vi "WPI_CANJaguar_GetVersion.vi"(8 "error in (no error)":errorcluster, 11 "CAN Jaguar Ref":T1={"DeviceStatus"={"status"=FALSE, "code"=0, "source"=""}, "Type"=enum."PWM", "PWM"={"PWM Channel"=enum."PWM 1", "DeadBand"={"Name"="", "maxPositivePwm"=0, "minPositivePwm"=0, "centerPwm"=0, "maxNegativePwm"=0, "minNegativePwm"=0, "angularRange"=0}}, "CAN"={"Device Number"=0, "SetOutput VI Ref"=variant(enum8{"Percent VBus", "Current", "Speed", "Position", "Voltage"} enum."Percent VBus"), "GetOutput VI Ref"=variant(refnum<k1> refnum), "Enable VI Ref"=variant(dbl 12.0), "Disable VI Ref"=variant(enum8{"Percent VBus", "Speed", "Position", "Slave", "Unchanged / Invalid", "Voltage Compensation", "Current", "Motion Profile"} enum."Percent VBus"), "Data"=variant}, "Invert"=FALSE}) -> (0 "error out":errorcluster, 1 "Hardware Version":u8, 2 "Firmware Version":u32, 3 "CAN Jaguar Ref Out":T1={"DeviceStatus"={"status"=FALSE, "code"=0, "source"=""}, "Type"=enum."PWM", "PWM"={"PWM Channel"=enum."PWM 1", "DeadBand"={"Name"="", "maxPositivePwm"=0, "minPositivePwm"=0, "centerPwm"=0, "maxNegativePwm"=0, "minNegativePwm"=0, "angularRange"=0}}, "CAN"={"Device Number"=0, "SetOutput VI Ref"=variant(enum8{"Percent VBus", "Current", "Speed", "Position", "Voltage"} enum."Percent VBus"), "GetOutput VI Ref"=variant(refnum<k1> refnum), "Enable VI Ref"=variant(dbl 12.0), "Disable VI Ref"=variant(enum8{"Percent VBus", "Speed", "Position", "Slave", "Unchanged / Invalid", "Voltage Compensation", "Current", "Motion Profile"} enum."Percent VBus"), "Data"=variant}, "Invert"=FALSE})   [LabVIEW 2016]
uses:
  <vilib>/Rock Robotics/WPI/MotorControl/WPI_MotorControlDeviceRef.ctl
  <vilib>/Rock Robotics/WPI/MotorControl/WPI_MotorControlType.ctl
  <vilib>/Rock Robotics/SystemInterfaces/DIO/FPGA_DIOPWMChannel.ctl
  <vilib>/Rock Robotics/WPI/PWM/WPI_PWMDeadband.ctl
  <vilib>/Rock Robotics/WPI/ThirdParty/CanMotor/CAN Jaguar/SubVIs/WPI_CAN_SystemMessageIDs.ctl
  <vilib>/Rock Robotics/WPI/ThirdParty/CanMotor/CAN Jaguar/SubVIs/WPI_CAN_UpdateMessageIDs.ctl
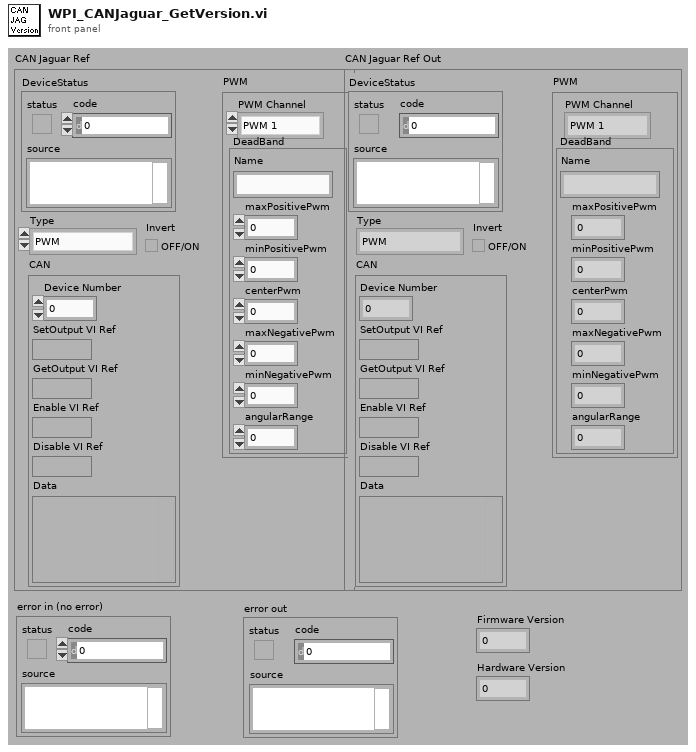
[diagram p1: front panel]
types:
  T1 = typedef "WPI_MotorControlDeviceRef.ctl" = cluster{"DeviceStatus":errorcluster, "Type":T2, "PWM":cluster{"PWM Channel":T3, "DeadBand":T4}, "CAN":cluster{"Device Number":u8, "SetOutput VI Ref":variant, "GetOutput VI Ref":variant, "Enable VI Ref":variant, "Disable VI Ref":variant, "Data":variant}, "Invert":bool}
  T2 = typedef "WPI_MotorControlType.ctl" = enum16{"PWM", "CAN"}
  T3 = typedef "FPGA_DIOPWMChannel.ctl" = enum8{"PWM 0", "PWM 1", "PWM 2", "PWM 3", "PWM 4", "PWM 5", "PWM 6", "PWM 7", "PWM 8", "PWM 9", "PWM MXP 0", "PWM MXP 1", "PWM MXP 2", "PWM MXP 3", "PWM MXP 4", "PWM MXP 5", "PWM MXP 6", "PWM MXP 7", "PWM MXP 8", "PWM MXP 9", "Invalid"}
  T4 = typedef "WPI_PWMDeadband.ctl" = cluster{"Name":string, "maxPositivePwm":i32, "minPositivePwm":i32, "centerPwm":i32, "maxNegativePwm":i32, "minNegativePwm":i32, "angularRange":u16}
  T5 = enum16{"big-endian, network order", "native, host order", "little-endian"}
  T6 = typedef "WPI_CAN_SystemMessageIDs.ctl" = u32
  T7 = typedef "WPI_CAN_UpdateMessageIDs.ctl" = u32
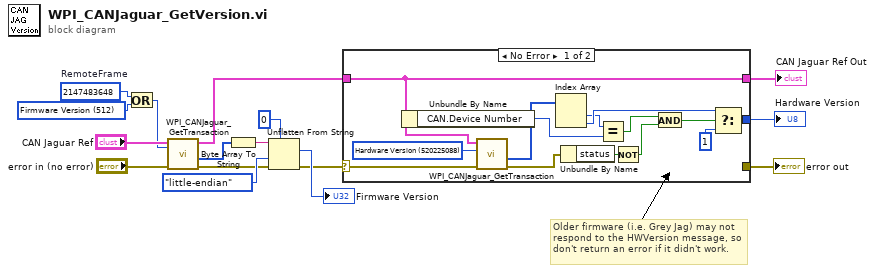
[diagram p0: block diagram]
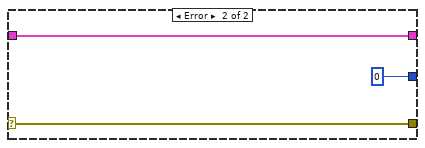
[diagram p2: hidden frame]
diagram:
  w1 = u32 2147483648  # RemoteFrame
  w8 = T6 512 items=["Device Assignment"=128, "Device Query"=192, "Sync Update"=384, "Firmware Update"=448, "Firmware Version"=512, "Enumerate"=576] ("CAN System Message IDs")
  # "Older firmware (i.e. Grey Jag) may not respond to the HWVersion message, so don't return an error if it didn't work."
  n1 = Or(x=w1, y=w8) -> (x .or. y?=w2:T6)
  n2 = call <vilib>:"WPI_CANJaguar_GetTransaction.vi"("error in"="error in (no error)", "Message ID"=w2, "CAN Jaguar Ref"="CAN Jaguar Ref") -> ("error out"=w6:errorcluster, "Data Out"=w3:u8[], "CAN Jaguar Ref Out"=w5:T1)  [unwired: 6 out]
  n3 = Byte Array To String(unsigned byte array=w3) -> (string=w16:string)
  n4 = Unflatten From String(type=u32 0, binary string=w16, byte order (0:big-endian, network order)=T5."little-endian", error in (no error)=w6) -> (value=→"Firmware Version":u32, error out=w10:errorcluster)  [unwired: 2 out]
  n5 = case shown="No Error" w10 {
    selector: w10 -> [w21 w33]
    tunnel: [_ w33] -> w12
    tunnel: [w26 u8 0 ("f")] -> w11
    tunnel: w5 -> [w18 w31]
    tunnel: [w18 w31] -> w4
    frame No Error {
      w22 = T7 520225088 items=["Update Ping"=520224768, "Update Download"=520224832, "Update Send Data"=520224896, "Update Reset"=520224960, "Update Acknowledge"=520225024, "Hardware Version"=520225088] ("CAN Update Message IDs")
      n6 = Unbundle By Name(w18) -> ("CAN.Device Number"=w17:u8)
      n7 = call <vilib>:"WPI_CANJaguar_GetTransaction.vi"("error in"=w21, "Message ID"=w22, "CAN Jaguar Ref"=w18) -> ("error out"=w20:errorcluster, "Data Out"=w19:u8[])  [unwired: 7 out]
      n8 = Index Array(array=w19) -> (element #1=w29:u8, element #2=w30:u8)  [unwired: 2 in]
      n9 = Unbundle By Name(w20) -> ("status"=w25:bool)
      n10 = Equal?(x=w29, y=w17) -> (x = y?=w28:bool)
      n11 = Not(x=w25) -> (.not. x?=w23:bool)
      n12 = And(x=w28, y=w23) -> (x .and. y?=w24:bool)
      n13 = Select(t=w30, s=w24, f=u8 1) -> (s? t:f=w26:u8)
    }
    frame Error {
    }
  }
  "error out" <- w12
  "Hardware Version" <- w11
  "CAN Jaguar Ref Out" <- w4
